vi "Init_DAQ_AI.vi"(8 "error in (no error)":errorcluster, 11 "Prueba21_1 in":refnum<class "Prueba21.lvclass">) -> (0 "error out":errorcluster, 3 "Prueba21_1 out":refnum<class "Prueba21.lvclass">)   [LabVIEW 2019, in "Prueba21.lvclass"]
uses:
  Prueba21.lvclass
  Prueba21.lvclass/Prueba21.ctl
  <vilib>/DAQmx/create/channels.llb/DAQmx Create Channel (AI-Voltage-Basic).vi
  <vilib>/DAQmx/configure/timing.llb/DAQmx Timing (Sample Clock).vi
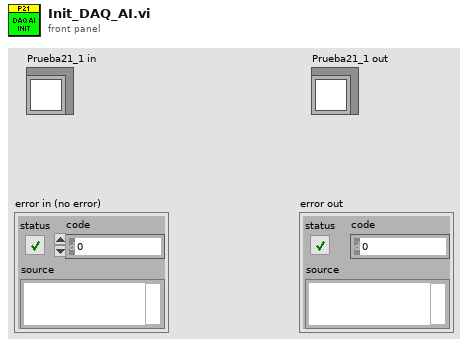
[diagram p1: front panel]
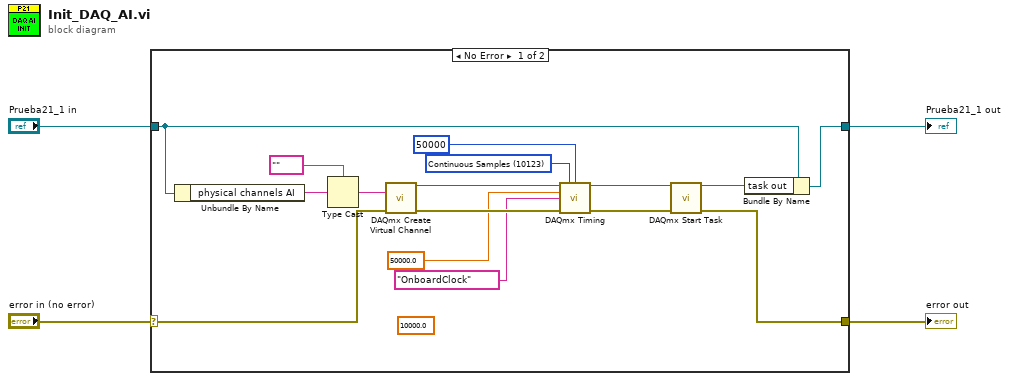
[diagram p0: block diagram]
diagram:
  n1 = case shown="No Error" "error in (no error)" {
    selector: "error in (no error)" -> [w17 w22]
    tunnel: [w14 w22] -> w2
    tunnel: [w15 w21] -> w3
    tunnel: "Prueba21_1 in" -> [w16 w21]
    frame No Error {
      (unwired) 10000.0 ("rate")
      w8 = 10123 items=["Finite Samples"=10178, "Continuous Samples"=10123, "Hardware Timed Single Point"=12522] ("sample mode")
      n2 = Unbundle By Name(w16) -> ("physical channels AI"=w20:string)
      n3 = Type Cast(type=tag "" ("physical channels"), x=w20) -> (*(type *) &x=w18:tag)
      n4 = call-poly <vilib>:"DAQmx Create Virtual Channel.vi"("physical channels"=w18, "error in"=w17) -> ("task out"=w11:refnum<k21>, "error out"=w13:errorcluster)  [unwired: 12 in]
      n5 = call-poly <vilib>:"DAQmx Timing.vi"("task/channels in"=w11, "sample mode"=w8, "samples per channel"=50000, "rate"=50000.0, "source"=tag "OnboardClock", "error in"=w13) -> ("task out"=w10:refnum<k21>, "error out"=w12:errorcluster)  [unwired: 8 in]
      n6 = call <vilib>:"DAQmx Start Task.vi"("task/channels in"=w10, "error in"=w12) -> ("task out"=w5:refnum<k21>, "error out"=w14:errorcluster)  [unwired: 12 in]
      n7 = Bundle By Name(cluster=w16, "task out"=w5) -> (w15:refnum<class "Prueba21.lvclass">)
    }
    frame Error {
    }
  }
  "Prueba21_1 out" <- w3
  "error out" <- w2
